vi "Calibrate.vi"(8 "error in (no error)":errorcluster, 11 "input":string) -> (0 "error out":errorcluster, 3 "blob":u8[](array[numeric]))   [LabVIEW 2015]
uses:
  C:/Distributed/CalFlex.dll
  CalFlex.dll
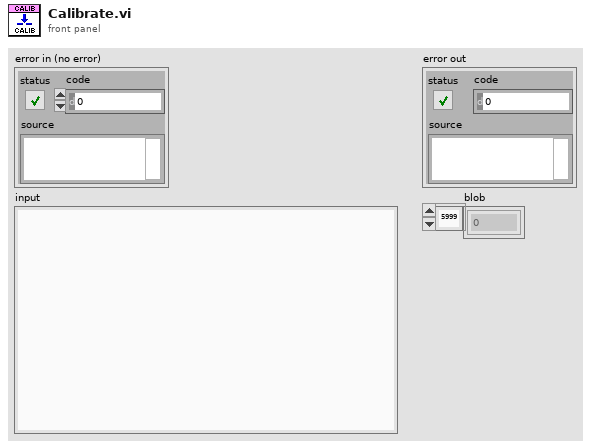
[diagram p1: front panel]
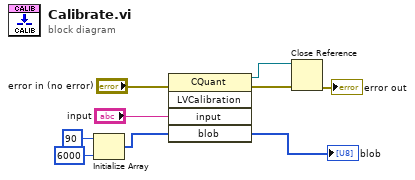
[diagram p0: block diagram]
diagram:
  n1 = Initialize Array(u8 90 ("dimension size"), 6000 ("dimension size")) -> (w2:u8[])
  n2 = invoke class="CQuant" method="LVCalibration"(error in="error in (no error)", "input"="input", "blob"=w2) -> (reference out=w6:refnum<k24>, error out=w7:errorcluster, "blob"=→"blob":u8[])  [unwired: 2 in, 2 out]
  n3 = Close Reference(reference=w6, error in (no error)=w7) -> (error out=→"error out":errorcluster)
